vi "Create.vi"(8 "error in (no error)":errorcluster, 11 "MB in":refnum<class "Master CR.lvclass">) -> (0 "error out":errorcluster, 3 "MB out":refnum<class "Master CR.lvclass">)   [LabVIEW 2021, in "Master CR.lvclass"]
uses:
  Master CR.lvclass
  Master CR.lvclass/Master CR.ctl
  ctl/CR_Core_State.ctl
  ctl/Master CR state.ctl
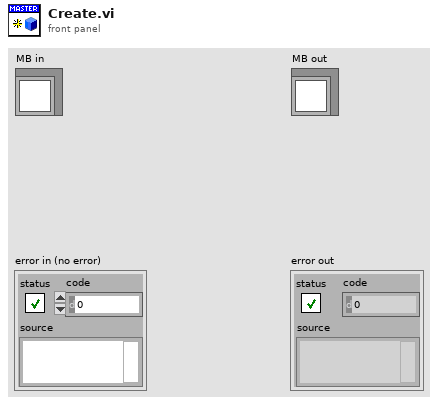
[diagram p1: front panel]
types:
  T1 = typedef "Master CR.lvclass/Master CR state.ctl" = cluster{"state":T2, "enable":bool, "write enable":bool, "connect":bool, "errors":i32, "Run":bool, "Write":bool, "Stop":bool}
  T2 = typedef "Master CR.lvclass/CR_Core_State.ctl" = enum8{"initialization", "redefine", "standby", "ping", "connect", "wait to reconnect", "wait to reset timeout", "configure", "requests", "close connection", "stop"}
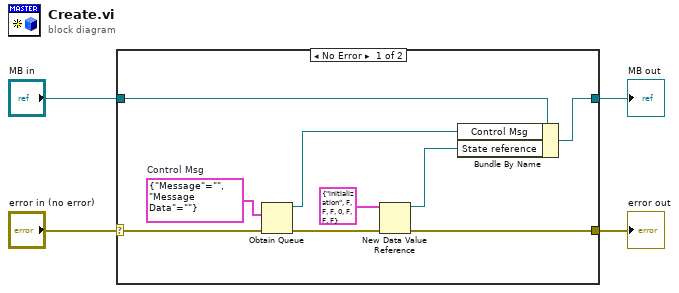
[diagram p0: block diagram]
diagram:
  n1 = case shown="No Error" "error in (no error)" {
    selector: "error in (no error)" -> [w6 w14]
    tunnel: "MB in" -> [w8 w15]
    tunnel: [w5 w14] -> w3
    tunnel: [w7 w15] -> w2
    frame No Error {
      w13 = cluster{"Message":string, "Message Data":string} {"Message"="", "Message Data"=""}  # Control Msg
      n2 = Obtain Queue(element data type=w13, error in (no error)=w6) -> (queue out=w10:refnum<queue>, error out=w9:errorcluster)  [unwired: 3 in, 1 out]
      n3 = New Data Value Reference(data value=T1 {"state"=enum."initialization", "enable"=FALSE, "write enable"=FALSE, "connect"=FALSE, "errors"=0, "Run"=FALSE, "Write"=FALSE, "Stop"=FALSE} ("State"), error in=w9) -> (data value reference=w11:refnum<data-value>, error out=w5:errorcluster)
      n4 = Bundle By Name(cluster=w8, "Control Msg"=w10, "State reference"=w11) -> (w7:refnum<class "Master CR.lvclass">)
    }
    frame Error {
    }
  }
  "error out" <- w3
  "MB out" <- w2
